vi "write_attributes.vi"(8 "error in (no error)":errorcluster, 10 "attributes":T1, 11 "SpectralEmbedding in":refnum<class "SpectralEmbedding.lvclass">) -> (0 "error out":errorcluster, 3 "SpectralEmbedding out":refnum<class "SpectralEmbedding.lvclass">)   [LabVIEW 2020, in "SpectralEmbedding.lvclass"]
uses:
  SpectralEmbedding.lvclass
  Controls/spectral_embedding_attributes.ctl
  SpectralEmbedding.lvclass/SpectralEmbedding.ctl
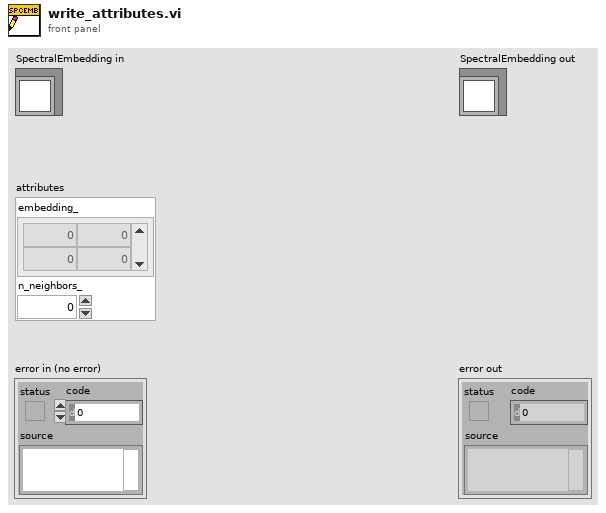
[diagram p1: front panel]
types:
  T1 = typedef "spectral_embedding_attributes.ctl" = cluster{"embedding_":dbl[][], "n_neighbors_":dbl}
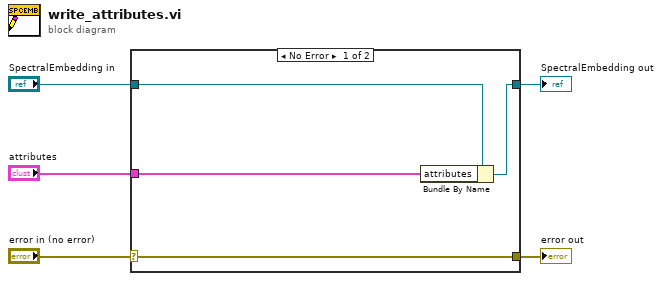
[diagram p0: block diagram]
diagram:
  n1 = case shown="No Error" "error in (no error)" {
    selector: "error in (no error)" -> [w9 w10]
    tunnel: [w9 w10] -> w4
    tunnel: [w7 w11] -> w2
    tunnel: "SpectralEmbedding in" -> [w8 w11]
    tunnel: "attributes" -> [w6 _]
    frame No Error {
      n2 = Bundle By Name(cluster=w8, "attributes"=w6) -> (w7:refnum<class "SpectralEmbedding.lvclass">)
    }
    frame Error {
    }
  }
  "error out" <- w4
  "SpectralEmbedding out" <- w2
